vi "cplx_to_string.vi"(1 "suffix (empty)":string, 2 "prefix (empty)":string, 3 "format string":string="%.6f", 4 "cplx in":cdb) -> (0 "formated string":string)   [LabVIEW 2013, in "varilib.lvlib"]
doc: "Somewhat prettier formatting of a complex number to string."
uses:
  varilib.lvlib
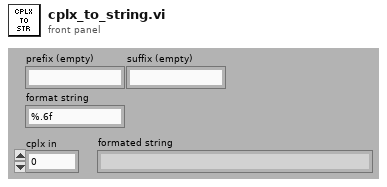
[diagram p1: front panel]
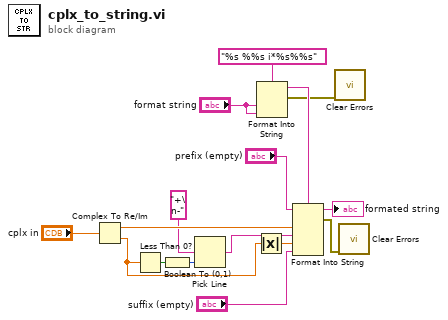
[diagram p0: block diagram]
diagram:
  n1 = Complex To Re/Im(x + iy="cplx in") -> (x=w14:dbl, y=w11:dbl)
  n2 = Less Than 0?(x=w11) -> (x < 0?=w13:bool)
  n3 = Boolean To (0,1)(Boolean=w13) -> (0, 1=w12:i16)
  n4 = Pick Line(multi-line string="+\n-", line index=w12) -> (output string=w15:string)  [unwired: 1 in]
  n5 = Absolute Value(x=w11) -> (abs(x)=w16:dbl)
  n6 = Format Into String(format string="%s %%s i*%s%%s", "format string", "format string") -> (resulting string=w5:string, error out=w2:errorcluster)  [unwired: 2 in]
  n7 = Format Into String(format string=w5, initial string="prefix (empty)", w14, w15, w16, "suffix (empty)") -> (resulting string=→"formated string":string, error out=w1:errorcluster)  [unwired: 1 in]
  n8 = call <vilib>:"Clear Errors.vi"("error in (no error)"=w2) -> ()  [unwired: 6 in, 1 out]
  n9 = call <vilib>:"Clear Errors.vi"("error in (no error)"=w1) -> ()  [unwired: 6 in, 1 out]
